vi "例6_下载EtherCat配置文件.vi"() -> ()   [LabVIEW 2012]
panel:
  in  "2.下载ENI文件路径":path
  in  "1.下载配置文件路径":path
  in  "初始值复位":bool
  in  "1.下载配置文件":bool
  in  "2.下载ENI文件":bool
  in  "使能关":bool
  in  "使能开":bool
  in  "硬复位":bool
  in  "软复位":bool
  out "复位提示":string
  out "总线状态":string
  out "当前速度":dbl
  in  "退出":bool
  in  "卡号选择":u16
  out "init":bool
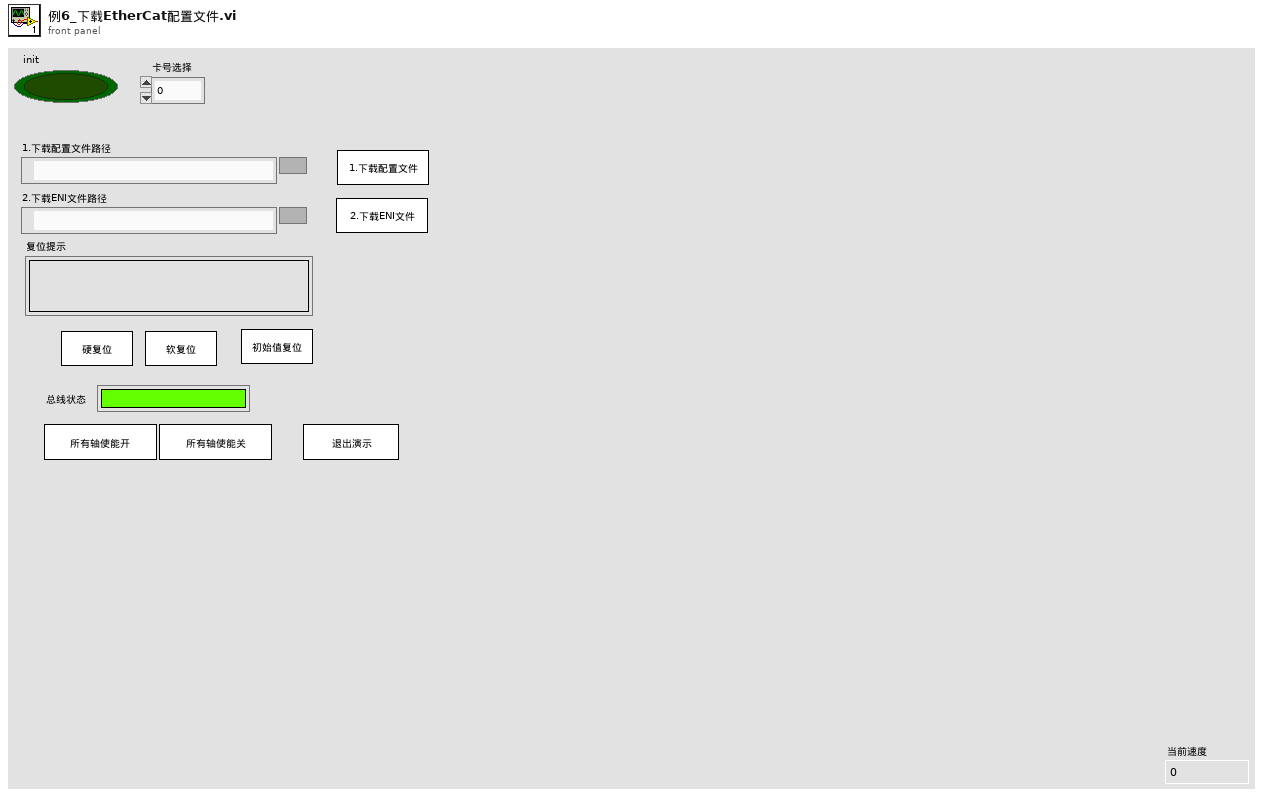
[diagram p1: front panel]
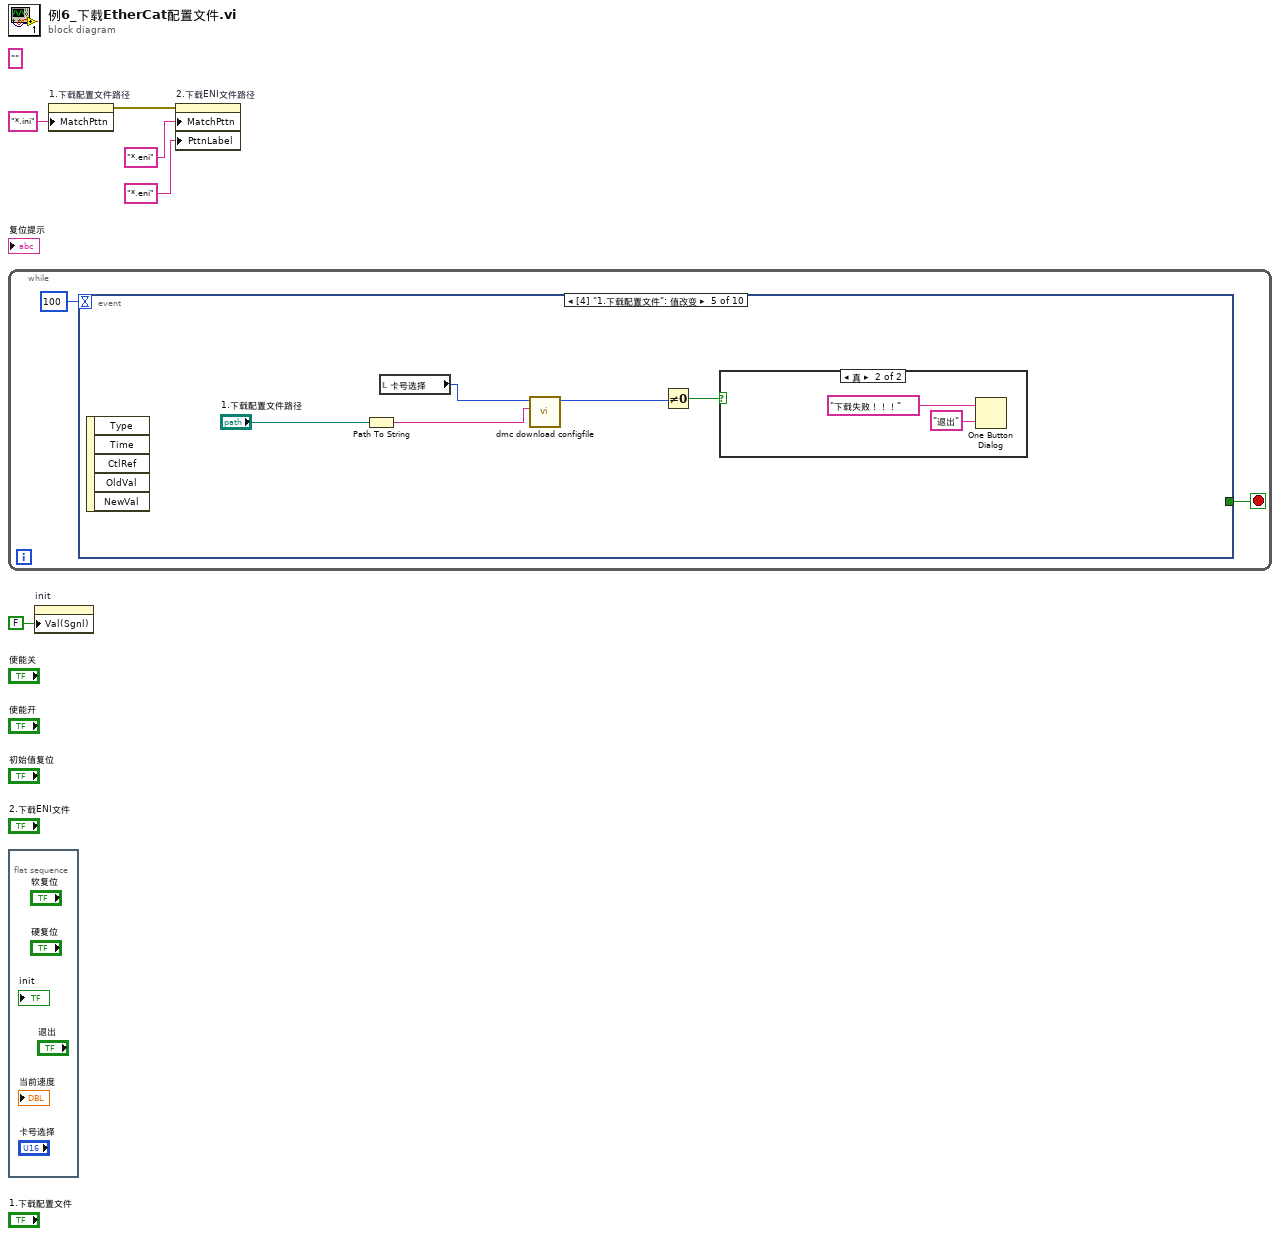
[diagram p0: block diagram]
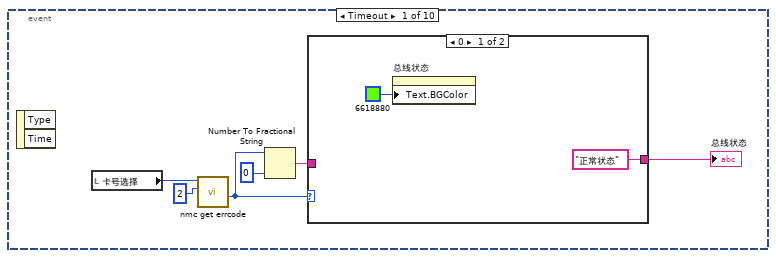
[diagram p2: hidden frame]
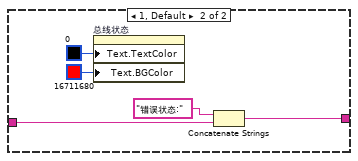
[diagram p3: hidden frame]
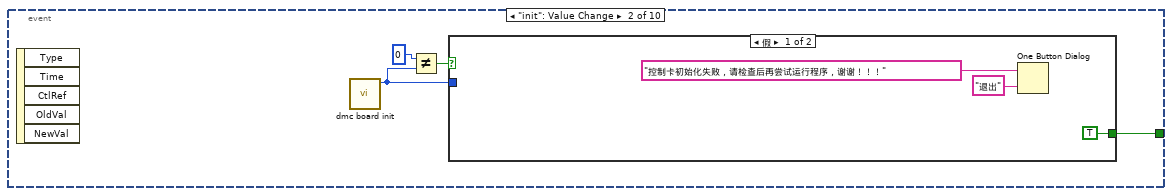
[diagram p4: hidden frame]
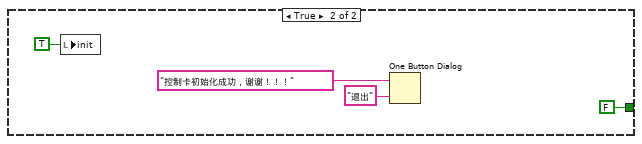
[diagram p5: hidden frame]
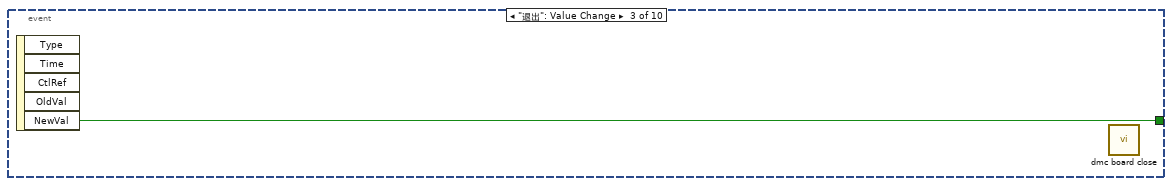
[diagram p6: hidden frame]
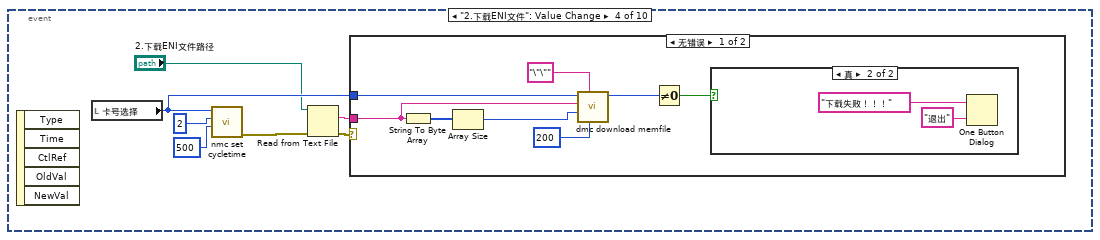
[diagram p7: hidden frame]
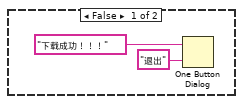
[diagram p8: hidden frame]
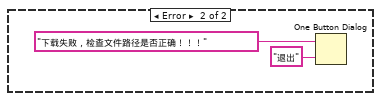
[diagram p9: hidden frame]
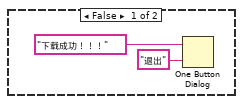
[diagram p10: hidden frame]
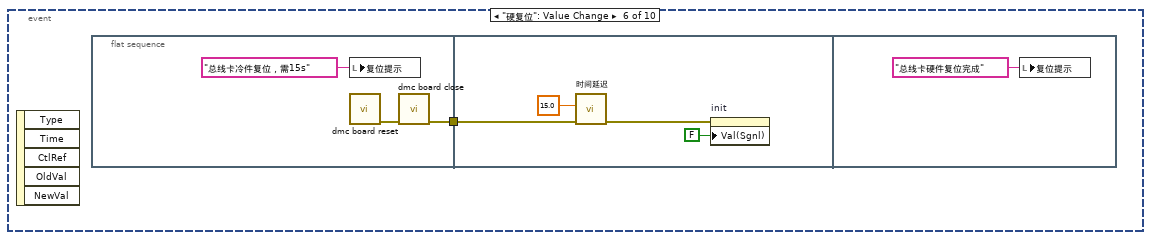
[diagram p11: hidden frame]
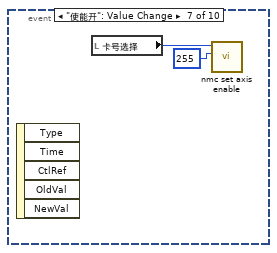
[diagram p12: hidden frame]
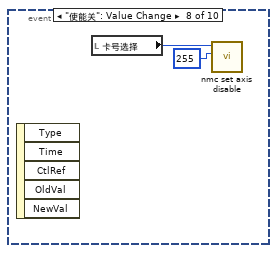
[diagram p13: hidden frame]
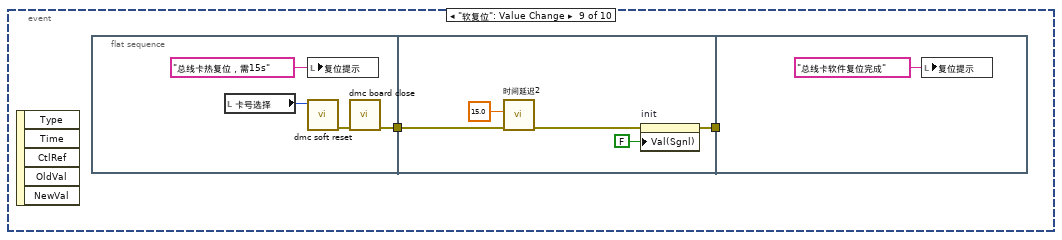
[diagram p14: hidden frame]
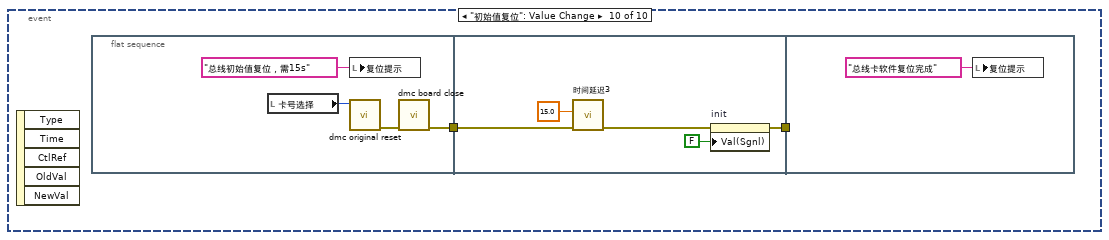
[diagram p15: hidden frame]
diagram:
  (unwired) "" ("浏览选项:类型标签")
  n1 = while {
    stop <- w7 stop-if-true
    n2 = event shown="[4] \"1.下载配置文件\": 值改变" {
      selector: _ -> [_ _ _ _ _ _ _ _ _ _]
      dyn-events: _ -> [_ _ _ _ _ _ _ _ _ _]
      timeout: 100 -> [_ _ _ _ _ _ _ _ _ _]
      tunnel: [_ w23 w32 _ _ _ _ _ _ _] -> w7
      event Timeout {
        n3 = event-data() -> ()  [unwired: 1 in, 2 out]
        n4 = local read "卡号选择"() -> (w8:u16)
        n5 = call "nmc get errcode.vi"("channel"=u16 2, "CardNo"=w8) -> ("Errcode out"=w10:u16)  [unwired: 7 in, 2 out]
        n6 = Number To Fractional String(number=w10, precision (6)=i16 0 ("精度(6)")) -> (F-format string=w9:string)  [unwired: 2 in]
        n7 = case shown="0" w10 {
          tunnel: ["正常状态" ("轴状态机") w18] -> w13
          tunnel: w9 -> [_ w19]
          frame 0 {
            n8 = property on="总线状态" class="Str"("Text.BGColor"=u32 6618880) -> ()  [unwired: 2 in, 2 out]
          }
          frame 1, Default {
            n9 = property on="总线状态" class="Str"("Text.TextColor"=u32 0, "Text.BGColor"=u32 16711680) -> ()  [unwired: 2 in, 2 out]
            n10 = Concatenate Strings("错误状态:" ("轴状态机"), w19) -> (w18:string)
          }
        }
        "总线状态" <- w13
      }
      event "init": Value Change {
        n11 = event-data() -> ()  [unwired: 1 in, 5 out]
        n12 = call "dmc board init.vi"() -> ("function return"=w22:i16)  [unwired: 10 in, 1 out]
        n13 = Not Equal?(x=0, y=w22) -> (x != y?=w24:bool)
        n14 = case shown="假" w24 {
          tunnel: [TRUE ("true") FALSE ("true")] -> w23
          tunnel: w22 -> [_ _]
          frame False {
            n15 = One Button Dialog(message="控制卡初始化失败，请检查后再尝试运行程序，谢谢！！！" ("消息"), button name ("OK")="退出" ("按钮名称（“确定”）")) -> ()  [unwired: 1 out]
          }
          frame True {
            n16 = local write "init"(TRUE ("init")) -> ()
            n17 = One Button Dialog(message="控制卡初始化成功，谢谢！！！" ("消息"), button name ("OK")="退出" ("按钮名称（“确定”）")) -> ()  [unwired: 1 out]
          }
        }
      }
      event "退出": Value Change {
        n18 = event-data() -> ("NewVal"=w32:bool)  [unwired: 1 in, 4 out]
        n19 = call "dmc board close.vi"() -> ()  [unwired: 10 in, 2 out]
      }
      event "2.下载ENI文件": Value Change {
        n20 = event-data() -> ()  [unwired: 1 in, 5 out]
        n21 = local read "卡号选择"() -> (w35:u16)
        n22 = call "nmc set cycletime.vi"("CycleTime"=u32 500, "PortNum"=u16 2, "CardNo"=w35) -> ("error out"=w34:errorcluster)  [unwired: 7 in, 1 out]
        n23 = Read from Text File(file (use dialog)="2.下载ENI文件路径", error in=w34) -> (text=w37:string, error out=w36:errorcluster)  [unwired: 2 in, 2 out]
        n24 = case shown="无错误" w36 {
          tunnel: w37 -> [w40 _]
          tunnel: w35 -> [w43 _]
          frame No Error {
            n25 = String To Byte Array(string=w40) -> (unsigned byte array=w42:u8[])
            n26 = Array Size(array=w42) -> (size(s)=w46:i32)
            n27 = call "dmc download memfile.vi"("filetype"=u16 200, "pfilenameinControl"="\"\"", "buffsize"=w46, "buffer"=w40, "CardNo"=w43) -> ("function return"=w44:i16)  [unwired: 4 in, 2 out]
            n28 = Not Equal To 0?(x=w44) -> (x != 0?=w45:bool)
            n29 = case shown="真" w45 {
              frame False {
                n30 = One Button Dialog(message="下载成功！！！" ("消息"), button name ("OK")="退出" ("按钮名称（“确定”）")) -> ()  [unwired: 1 out]
              }
              frame True {
                n31 = One Button Dialog(message="下载失败！！！" ("消息"), button name ("OK")="退出" ("按钮名称（“确定”）")) -> ()  [unwired: 1 out]
              }
            }
          }
          frame Error {
            n32 = One Button Dialog(message="下载失败，检查文件路径是否正确！！！" ("消息"), button name ("OK")="退出" ("按钮名称（“确定”）")) -> ()  [unwired: 1 out]
          }
        }
      }
      event "1.下载配置文件": Value Change {
        n33 = event-data() -> ()  [unwired: 1 in, 5 out]
        n34 = Path To String(path="1.下载配置文件路径") -> (string=w56:string)
        n35 = local read "卡号选择"() -> (w57:u16)
        n36 = call "dmc download configfile.vi"("FileName"=w56, "CardNo"=w57) -> ("function return"=w54:i16)  [unwired: 8 in, 1 out]
        n37 = Not Equal To 0?(x=w54) -> (x != 0?=w55:bool)
        n38 = case shown="真" w55 {
          frame False {
            n39 = One Button Dialog(message="下载成功！！！" ("消息"), button name ("OK")="退出" ("按钮名称（“确定”）")) -> ()  [unwired: 1 out]
          }
          frame True {
            n40 = One Button Dialog(message="下载失败！！！" ("消息"), button name ("OK")="退出" ("按钮名称（“确定”）")) -> ()  [unwired: 1 out]
          }
        }
      }
      event "硬复位": Value Change {
        n41 = event-data() -> ()  [unwired: 1 in, 5 out]
        n42 = flat-sequence {
          tunnel: [w65] -> w63
          tunnel: w63 -> [w67]
          frame #0 {
            n43 = local write "复位提示"("总线卡冷件复位，需15s" ("运行提示")) -> ()
            n44 = call "dmc board reset.vi"() -> ("error out"=w66:errorcluster)  [unwired: 10 in, 1 out]
            n45 = call "dmc board close.vi"("error in (no error)"=w66) -> ("error out"=w65:errorcluster)  [unwired: 9 in, 1 out]
          }
          frame #1 {
            n46 = call "时间延迟"("error in (no error)"=w67, "Delay Time (s)"=15.0) -> ("error out"=w70:errorcluster)  [unwired: 9 in]
            n47 = property on="init" class="Bool (严格)"(error in=w70, "Val(Sgnl)"=FALSE ("值(信号)")) -> ()  [unwired: 1 in, 2 out]
          }
          frame #2 {
            n48 = local write "复位提示"("总线卡硬件复位完成" ("运行提示")) -> ()
          }
        }
      }
      event "使能开": Value Change {
        n49 = event-data() -> ()  [unwired: 1 in, 5 out]
        n50 = local read "卡号选择"() -> (w73:u16)
        n51 = call "nmc set axis enable.vi"("axis"=u16 255, "CardNo"=w73) -> ()  [unwired: 8 in, 2 out]
      }
      event "使能关": Value Change {
        n52 = event-data() -> ()  [unwired: 1 in, 5 out]
        n53 = local read "卡号选择"() -> (w75:u16)
        n54 = call "nmc set axis disable.vi"("axis"=u16 255, "CardNo"=w75) -> ()  [unwired: 8 in, 2 out]
      }
      event "软复位": Value Change {
        n55 = event-data() -> ()  [unwired: 1 in, 5 out]
        n56 = flat-sequence {
          tunnel: [w81] -> w77
          tunnel: w77 -> [w83]
          tunnel: [w82] -> w76
          tunnel: w76 -> [_]
          frame #0 {
            n57 = local read "卡号选择"() -> (w78:u16)
            n58 = local write "复位提示"("总线卡热复位，需15s" ("运行提示")) -> ()
            n59 = call "dmc soft reset.vi"("CardNo"=w78) -> ("error out"=w79:errorcluster)  [unwired: 9 in, 1 out]
            n60 = call "dmc board close.vi"("error in (no error)"=w79) -> ("error out"=w81:errorcluster)  [unwired: 9 in, 1 out]
          }
          frame #1 {
            n61 = call "时间延迟2"("error in (no error)"=w83, "Delay Time (s)"=15.0) -> ("error out"=w86:errorcluster)  [unwired: 9 in]
            n62 = property on="init" class="Bool (严格)"(error in=w86, "Val(Sgnl)"=FALSE ("值(信号)")) -> (error out=w82:errorcluster)  [unwired: 1 in, 1 out]
          }
          frame #2 {
            n63 = local write "复位提示"("总线卡软件复位完成" ("运行提示")) -> ()
          }
        }
      }
      event "初始值复位": Value Change {
        n64 = event-data() -> ()  [unwired: 1 in, 5 out]
        n65 = flat-sequence {
          tunnel: [w93] -> w89
          tunnel: w89 -> [w95]
          tunnel: [w94] -> w88
          tunnel: w88 -> [_]
          frame #0 {
            n66 = local read "卡号选择"() -> (w90:u16)
            n67 = local write "复位提示"("总线初始值复位，需15s" ("运行提示")) -> ()
            n68 = call "dmc original reset.vi"("CardNo"=w90) -> ("error out"=w91:errorcluster)  [unwired: 9 in, 1 out]
            n69 = call "dmc board close.vi"("error in (no error)"=w91) -> ("error out"=w93:errorcluster)  [unwired: 9 in, 1 out]
          }
          frame #1 {
            n70 = call "时间延迟3"("error in (no error)"=w95, "Delay Time (s)"=15.0) -> ("error out"=w98:errorcluster)  [unwired: 9 in]
            n71 = property on="init" class="Bool (严格)"(error in=w98, "Val(Sgnl)"=FALSE ("值(信号)")) -> (error out=w94:errorcluster)  [unwired: 1 in, 1 out]
          }
          frame #2 {
            n72 = local write "复位提示"("总线卡软件复位完成" ("运行提示")) -> ()
          }
        }
      }
    }
  }
  n73 = flat-sequence {
    frame #0 {
    }
  }
  n74 = property on="init" class="Bool (严格)"("Val(Sgnl)"=FALSE ("值(信号)")) -> ()  [unwired: 2 in, 2 out]
  n75 = property on="1.下载配置文件路径" class="Path"("MatchPttn"="*.ini" ("浏览选项:匹配模式")) -> (error out=w2:errorcluster)  [unwired: 2 in, 1 out]
  n76 = property on="2.下载ENI文件路径" class="Path"(error in=w2, "MatchPttn"="*.eni" ("浏览选项:匹配模式"), "PttnLabel"="*.eni" ("浏览选项:类型标签")) -> ()  [unwired: 1 in, 2 out]
